vi "LM 2D Gaussian ACF and gradient.vi"(3 "output control":T1, 4 "data":variant, 5 "X":dbl[](array[numeric]), 6 "a":dbl[](array[numeric])) -> (0 "error out":errorcluster, 1 "f'(X,a)":dbl[][](array[numeric]), 2 "f(X,a)":dbl[](array[numeric]))   [LabVIEW 2021, in "Fits.lvlib"]
doc: "This template is the starting point for creating a model function to be passed to the Nonlinear Curve Fit.vi."
uses:
  <vilib>/gmath/NumericalOptimization/LM_output select.ctl
  Fits.lvlib
  <vilib>/gmath/NI_Gmath.lvlib
panel:
  # "Parameters:\n\namplitude: A\ndiffusion time: t"
  # "f(x) = 1 + A/(1+x/t)"
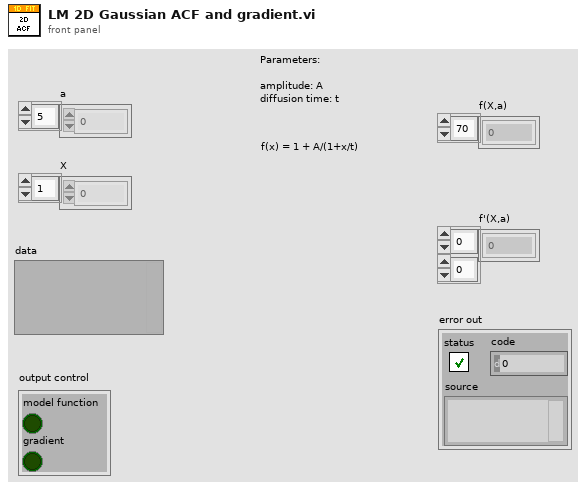
[diagram p1: front panel]
types:
  T1 = typedef "NI_Gmath.lvlib/LM_output select.ctl" = cluster{"model function":bool, "gradient":bool}
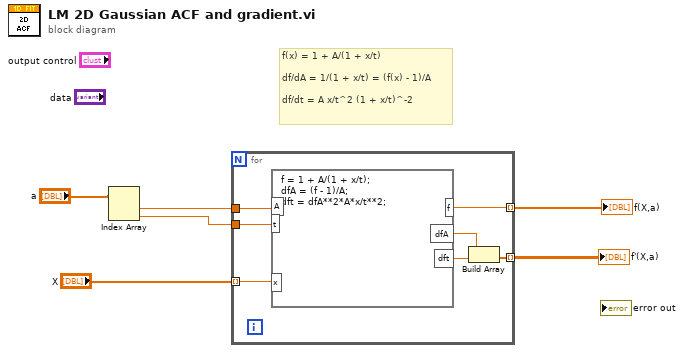
[diagram p0: block diagram]
diagram:
  # "f(x) = 1 + A/(1 + x/t)\n\ndf/dA = 1/(1 + x/t) = (f(x) - 1)/A\n\ndf/dt = A x/t^2 (1 + x/t)^-2"
  n1 = Index Array(array="a") -> (element #1=w2:dbl, element #2=w1:dbl)  [unwired: 2 in]
  n2 = for {
    tunnel: w2 -> [w12]
    tunnel: w1 -> [w13]
    tunnel: "X" -> [w11] mode=indexing
    tunnel: [w10] -> w4 mode=indexing
    tunnel: [w7] -> w3 mode=indexing
    n3 = formula code="f = 1 + A/(1 + x/t);\ndfA = (f - 1)/A;\ndft = dfA**2*A*x/t**2;"("A"=w12, "t"=w13, "x"=w11) -> ("f"=w10:dbl, "dfA"=w9:dbl, "dft"=w8:dbl)
    n4 = Build Array(w9, w8) -> (w7:dbl[])
  }
  "f(X,a)" <- w4
  "f'(X,a)" <- w3
